vi "Main VI with license checker.vi"() -> ()   [LabVIEW 2016]
panel:
  out "error out":errorcluster
  out "valid?":bool
  out "number (0 to 1)":dbl
  in  "stop":bool
  # "Generate a new license file with difference prefix text to see the behavior."
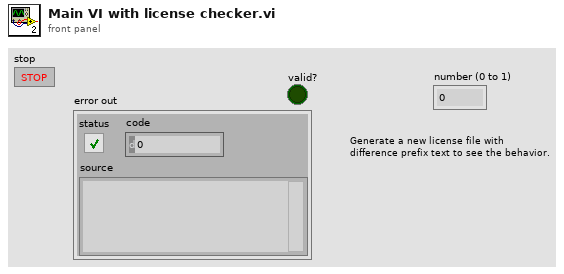
[diagram p1: front panel]
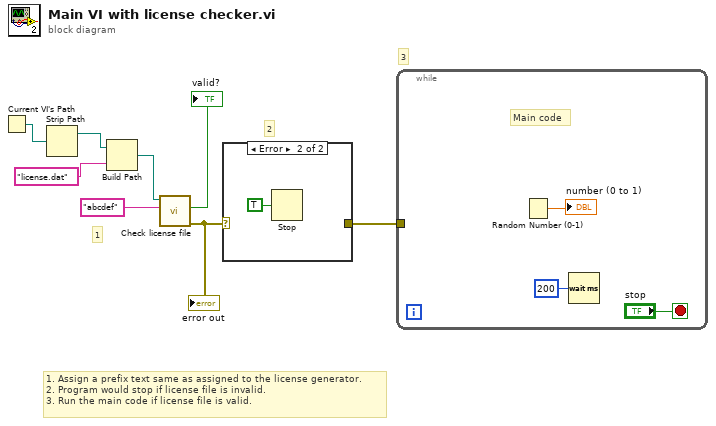
[diagram p0: block diagram]
diagram:
  # "3"
  # "2"
  # "1. Assign a prefix text same as assigned to the license generator. \n2. Program would stop if license file is invalid.\n3. Run the main code if license file is valid."
  # "1"
  n1 = Current VI's Path() -> (path=w4:path)
  n2 = Strip Path(path=w4) -> (stripped path=w3:path)  [unwired: 1 out]
  n3 = Build Path(base path=w3, name or relative path="license.dat") -> (appended path=w2:path)
  n4 = call "Check license file.vi"("prefix text"="abcdef", "file path"=w2) -> ("error out"=w7:errorcluster, "valid?"=→"valid?":bool)  [unwired: 7 in, 1 out]
  "error out" <- w7
  n5 = case shown="Error" w7 {
    selector: w7 -> [w9 _]
    tunnel: [w9 _] -> w6
    frame No Error {
    }
    frame Error {
      n6 = Stop(stop? (T)=TRUE) -> ()
    }
  }
  n7 = while {
    tunnel: w6 -> [_]
    stop <- "stop" stop-if-true
    # "Main code"
    n8 = Random Number (0-1)() -> (number: 0 to 1=→"number (0 to 1)":dbl)
    n9 = Wait (ms)(milliseconds to wait=u32 200) -> ()  [unwired: 1 out]
  }
